vi "Obtain shut down event.vi"(8 "error in (no error)":errorcluster) -> (0 "error out":errorcluster, 3 "Shut down":refnum<user-event>)   [LabVIEW 2018, in "Fiber Auto Collimation References.lvclass"]
doc: "This VI returns the reference to an event that will shut down all event handlers on the main VI, any panels running, (and possibly elsewhere, if any other asynchronous routines register for it).\n\nThis event is intended only to be triggered after the main Model loop has exited. Triggering it inside the Model loop or in SubVIs is not recommended.\n\nThe default behavior is that \"False\" shuts down loops that interact with controls and indicators (the \"View\" and \"Controller\" loops) while \"True\" shuts down everything, including those loops but also any others, notably the loop or loops that listen for the \"Kill process\" signal but also any others that may have been created."
uses:
  Fiber Auto Collimation References.lvclass
  C:/Program Files (x86)/National Instruments/LabVIEW 2018/user.lib/nLight Tidbits/Cross-library references/Cross-library key/Cross-library key.lvclass
  0922117a-040d-4c18-b692-367c81ced159.vi
  df0ec1d4-b4fd-4768-964e-08eeb2f8a793.vi
  0922117a-040d-4c18-b692-367c81ced159.vi/cce1f634-8d9a-4da1-a76c-12f7a8cb42cb.vi
  <userlib>/nLight Tidbits/Cross-library references/Cross-library key/Obtain cross library semaphore and acquire.vi
  0922117a-040d-4c18-b692-367c81ced159.vi/077d14da-6783-4c13-ac19-1b21dcec63b0.vi
  df0ec1d4-b4fd-4768-964e-08eeb2f8a793.vi/b37a6595-6989-434d-b56e-090d44e166e2.vi
  df0ec1d4-b4fd-4768-964e-08eeb2f8a793.vi/ac4bb57f-4b3b-434e-9121-c078f2b23829.vi
  <userlib>/nLight Error Handling/Trash error.vi
  <vilib>/Utility/error.llb/Clear Errors.vi
  <vilib>/Utility/semaphor.llb/Obtain Semaphore Reference.vi
  <vilib>/Utility/semaphor.llb/Acquire Semaphore.vi
  <userlib>/nLight Error Handling/Log any errors.vi
  <userlib>/nLight Tidbits/Cross-library references/Cross-library key/Obtain class key.vi
  <vilib>/Utility/semaphor.llb/Release Semaphore.vi
  <vilib>/Utility/semaphor.llb/Release Semaphore Reference.vi
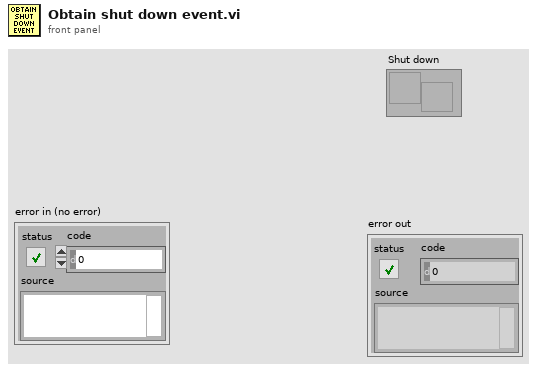
[diagram p1: front panel]
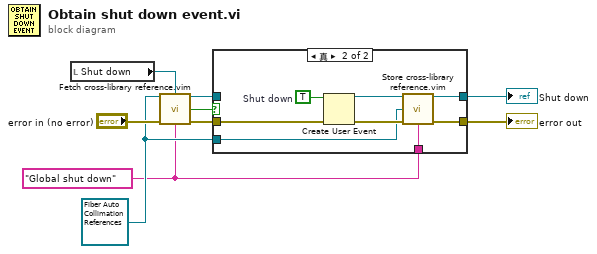
[diagram p0: block diagram]
diagram:
  w1 = "Global shut down"
  w4 = refnum<class "Fiber Auto Collimation References.lvclass"> refnum ("nLight Station Template References.lvclass")
  n1 = local read "Shut down"() -> (w5:refnum<user-event>)
  n2 = call "Fetch cross-library reference.vim"("Cross-library key"=w4, "Reference type to fetch"=w5, "error in (no error)"="error in (no error)", "Specific ref type name [String/Enum]"=w1) -> ("Stored value (if present)"=w2:refnum<user-event>, "Nothing to fetch OR bad reference"=w6:bool, "error out"=w7:errorcluster)  [unwired: 9 in]
  n3 = case shown="真" w6 {
    tunnel: w7 -> [w10 w19]
    tunnel: [w10 w16] -> w9
    tunnel: [w11 w14] -> w3
    tunnel: w2 -> [w11 _]
    tunnel: w4 -> [_ w13]
    tunnel: w1 -> [_ w12]
    frame False {
    }
    frame True {
      w18 = TRUE  # Shut down
      n4 = Create User Event(user event datatype=w18, error in=w19) -> (user event=w15:refnum<user-event>, error out=w17:errorcluster)
      n5 = call "Store cross-library reference.vim"("Reference to store"=w15, "Cross-library key"=w13, "error in (no error)"=w17, "Specific ref type name [String/Enum]"=w12) -> ("Copy of stored reference"=w14:refnum<user-event>, "error out"=w16:errorcluster)  [unwired: 8 in, 2 out]
    }
  }
  "error out" <- w9
  "Shut down" <- w3
